vi "programa 7.vi"() -> ()   [LabVIEW 2011]
panel:
  out "Array":T1(array[cluster]) {"velocidad 3" scale=0.0..180.0; "velocidad 2" scale=0.0..180.0; "velocidad" scale=0.0..180.0}
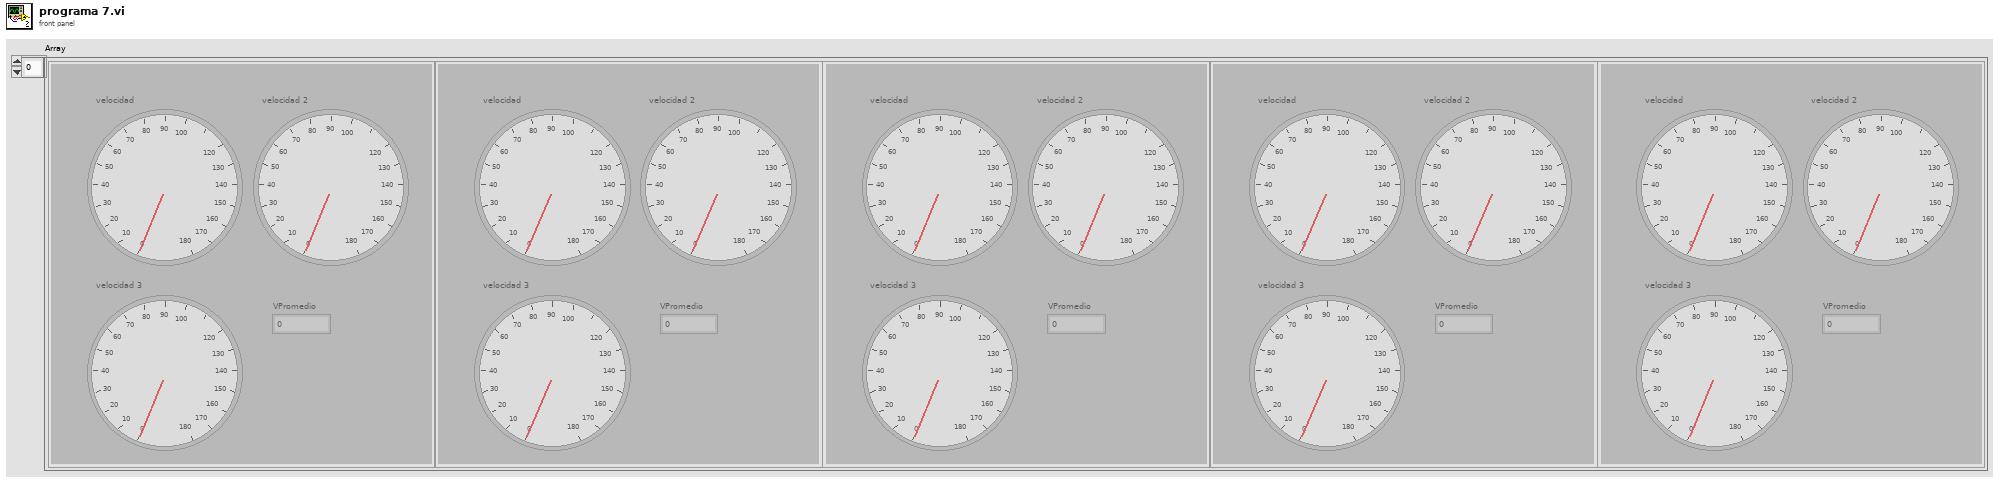
[diagram p1: front panel]
types:
  T1 = cluster{"velocidad":i32, "velocidad 2":i32, "velocidad 3":i32, "VPromedio":dbl}[]
  T2 = enum16{"open", "replace", "create", "open or create", "replace or create", "replace or create with confirmation"}
  T3 = cluster{"velocidad":i32, "velocidad 2":i32, "velocidad 3":i32, "VPromedio":dbl}
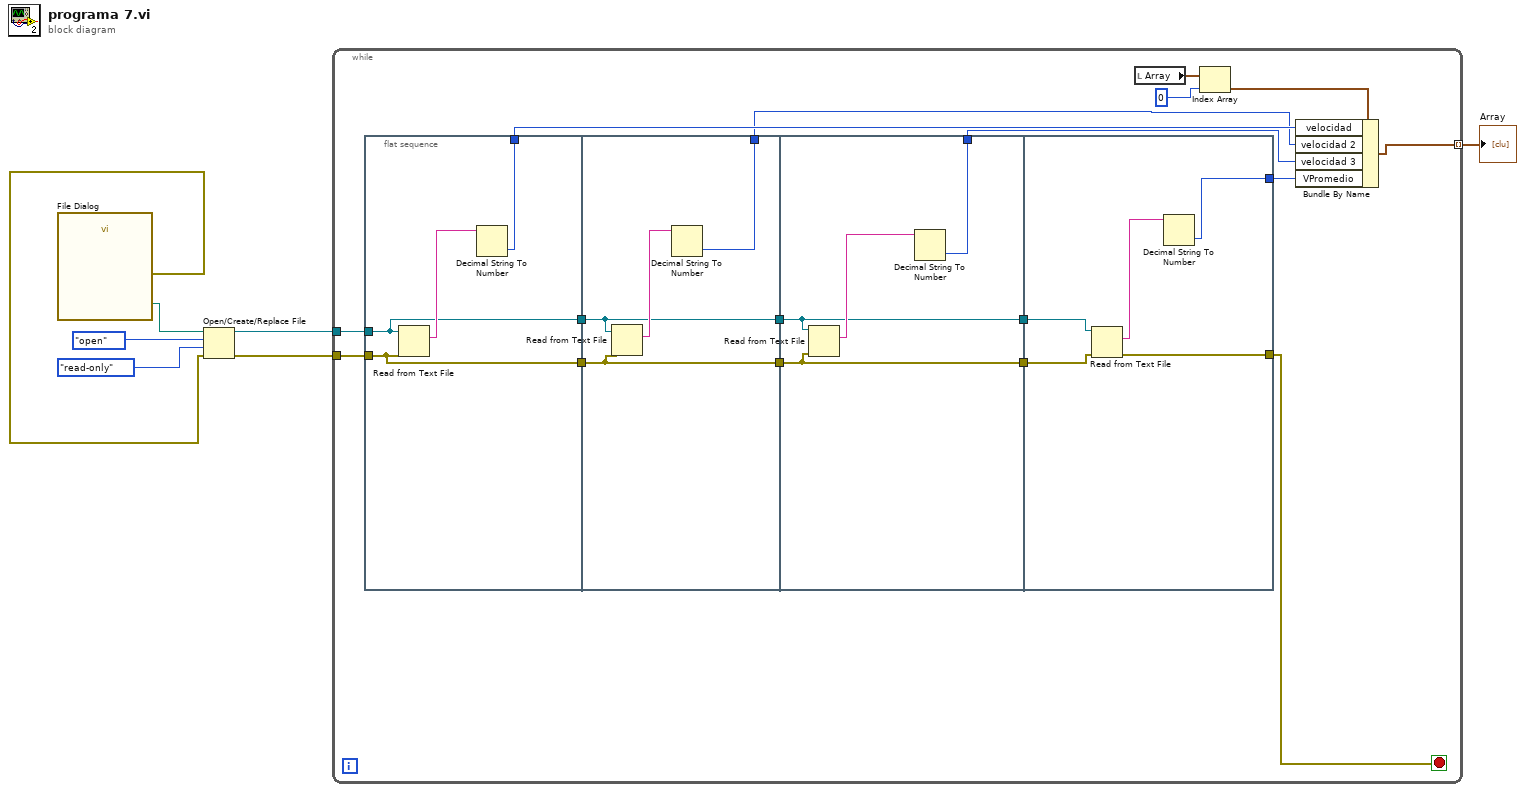
[diagram p0: block diagram]
diagram:
  n1 = call "File Dialog"() -> ("selected path"=w7:path, "error out"=w6:errorcluster)  [unwired: 12 in, 2 out]
  n2 = Open/Create/Replace File(file path (use dialog)=w7, error in=w6, operation (0:open)=T2."open", access (0:read/write)=enum16{"read/write", "read-only", "write-only"}."read-only") -> (refnum out=w3:refnum<file>, error out=w2:errorcluster)  [unwired: 2 in, 1 out]
  n3 = while {
    tunnel: w3 -> [w24]
    tunnel: w2 -> [w23]
    tunnel: [w8] -> w1 mode=indexing
    stop <- w9 stop-if-true
    n4 = flat-sequence {
      tunnel: w24 -> [w26]
      tunnel: w23 -> [w27]
      tunnel: [w27] -> w22
      tunnel: [w26] -> w21
      tunnel: [w25] -> w13
      tunnel: w22 -> [w31]
      tunnel: w21 -> [w30]
      tunnel: [w31] -> w20
      tunnel: [w30] -> w19
      tunnel: [w29] -> w12
      tunnel: w20 -> [w35]
      tunnel: w19 -> [w34]
      tunnel: [w35] -> w18
      tunnel: [w34] -> w17
      tunnel: [w33] -> w11
      tunnel: w18 -> [w41]
      tunnel: w17 -> [w40]
      tunnel: [w38] -> w10
      tunnel: [w37] -> w9
      frame #0 {
        n5 = Read from Text File(file (use dialog)=w26, error in=w27) -> (text=w28:string)  [unwired: 2 in, 3 out]
        n6 = Decimal String To Number(string=w28) -> (number=w25:i32)  [unwired: 2 in, 1 out]
      }
      frame #1 {
        n7 = Read from Text File(file (use dialog)=w30, error in=w31) -> (text=w32:string)  [unwired: 2 in, 3 out]
        n8 = Decimal String To Number(string=w32) -> (number=w29:i32)  [unwired: 2 in, 1 out]
      }
      frame #2 {
        n9 = Read from Text File(file (use dialog)=w34, error in=w35) -> (text=w36:string)  [unwired: 2 in, 3 out]
        n10 = Decimal String To Number(string=w36) -> (number=w33:i32)  [unwired: 2 in, 1 out]
      }
      frame #3 {
        n11 = Read from Text File(file (use dialog)=w40, error in=w41) -> (text=w39:string, error out=w37:errorcluster)  [unwired: 2 in, 2 out]
        n12 = Decimal String To Number(string=w39) -> (number=w38:i32)  [unwired: 2 in, 1 out]
      }
    }
    n13 = local read "Array"() -> (w16:T1)
    n14 = Index Array(array=w16, index=0) -> (element=w14:T3)
    n15 = Bundle By Name "Bundle By Name"(cluster=w14, "velocidad"=w13, "velocidad 2"=w12, "velocidad 3"=w11, "VPromedio"=w10) -> (w8:T3)
  }
  "Array" <- w1
